vi "Analyse.vi"(8 "error in (no error)":errorcluster, 10 "ImageData":T1, 11 "FluorescenceAnalyser in":refnum<class "FluorescenceAnalyser.lvclass">) -> (0 "error out":errorcluster, 3 "FluorescenceAnalyser out":refnum<class "FluorescenceAnalyser.lvclass">)   [LabVIEW 2009, in "Tools.lvlib" / "Imaging.lvlib" / "FluorescenceAnalyser.lvclass"]
uses:
  FluorescenceAnalyser.lvclass
  ImageAnalyser.lvclass
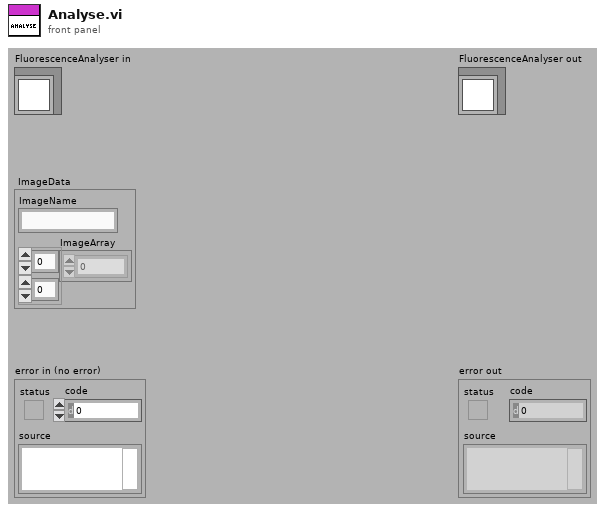
[diagram p1: front panel]
types:
  T1 = cluster{"ImageName":string, "ImageArray":sgl[][]}
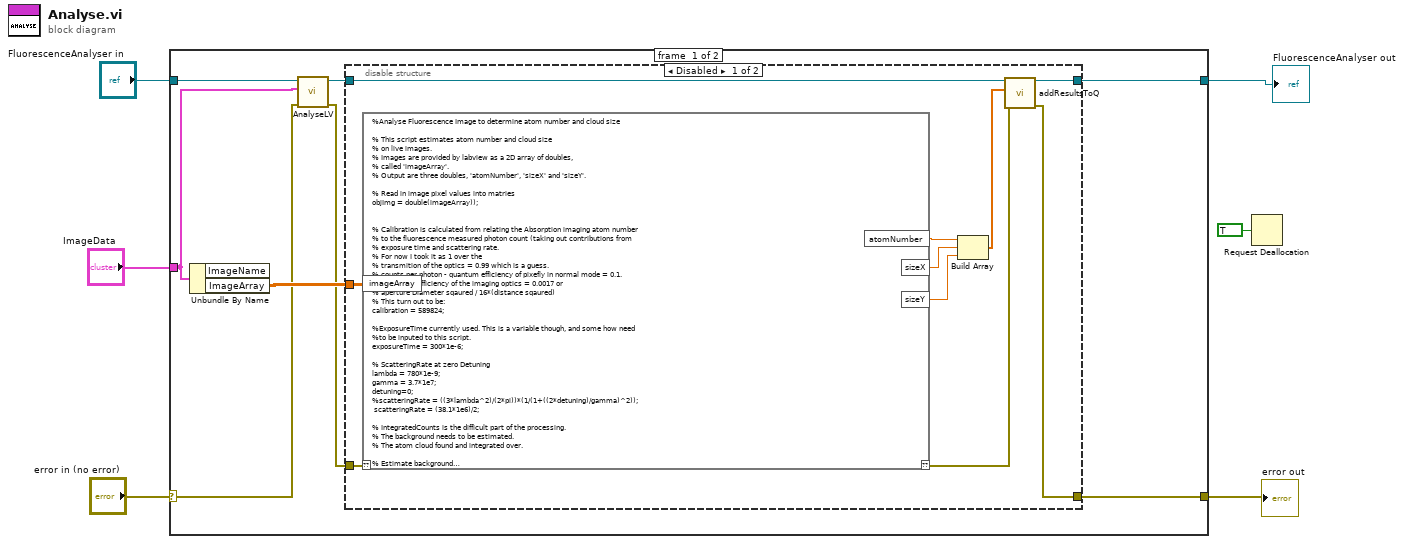
[diagram p0: block diagram]
diagram:
  n1 = case shown="No Error" "error in (no error)" {
    selector: "error in (no error)" -> [w8 w27]
    tunnel: "FluorescenceAnalyser in" -> [w11 w28]
    tunnel: "ImageData" -> [w10 _]
    tunnel: [w12 w27] -> w3
    tunnel: [w13 w28] -> w2
    frame #0 {
      n2 = Unbundle By Name(w10) -> ("ImageArray"=w14:sgl[][])  [unwired: 1 out]
      n3 = call "AnalyseLV.vi"("error in (no error)"=w8, "ImageData"=w10, "FluorescenceAnalyser in"=w11) -> ("error out"=w7:errorcluster, "FluorescenceAnalyser out"=w9:refnum<class "FluorescenceAnalyser.lvclass">)  [unwired: 7 in]
      n4 = disable-structure shown="Disabled" {
        disable-tunnel: w14 -> [w24 _]
        disable-tunnel: [w20 w26] -> w13
        disable-tunnel: [w19 w25] -> w12
        disable-tunnel: w7 -> [w17 w25]
        disable-tunnel: w9 -> [w16 w26]
        frame #0 {
          n5 = script code="%Analyse Fluorescence Image to determine atom number and cloud size\n\n% This script estimates atom number and cloud size\n% on live images. \n% Images are provided by labview as a 2D array of doubles,\n% called 'imageArray'.\n% Output are three doubles, 'atomNumber', 'sizeX' and 'sizeY'.\n\n% Read in image pixel values into matries\nobjImg = double(imageArray));\n\n\n% Calibration is calculated from relating the Absorption imaging atom number\n% to the fluorescence measured photon count (taking out contributions from\n% exposure time and scattering rate.\n% For now I took it as 1 over the \n% transmition of the optics = 0.99 which is a guess.\n% counts per photon - quantum efficiency of pixefly in normal mode = 0.1.\n% Collection efficiency of the imaging optics = 0.0017 or \n% aperture Diameter sqaured / 16*(distance sqaured)\n% This turn out to be:\ncalibration = 589824;\n\n%ExposureTime currently used. This is a variable though, and some how need\n%to be inputed to this script.\nexposureTime = 300*1e-6;\n\n% ScatteringRate at zero Detuning\nlambda = 780*1e-9;\ngamma = 3.7*1e7;\ndetuning=0;\n%scatteringRate = ((3*lambda^2)/(2*pi))*(1/(1+((2*detuning)/gamma)^2));\n scatteringRate = (38.1*1e6)/2;\n\n% IntegratedCounts is the difficult part of the processing.\n% The background needs to be estimated.\n% The atom cloud found and integrated over.\n\n% Estimate background \nbg = mean(mean(objImg(10,:)));\n\nimage = objImg-bg;\n\nintegratedCounts = sum(sum(image));\n%absimagecount=integratedCounts*scatteringRate/(6.45e-6)^2;\n%Calculate Atom number\natomNumber = ( calibration/(exposureTime*scatteringRate) )*integratedCounts;\n\n%subplot(3,2,1), imagesc(image(200:800,400:1000)), \n%subplot(3,2,2), plot(image(:,691));\n%subplot(3,2,3), plot(image(507,:));\n%axes('position',[0,0,1,1],'visible','off');\n%text(.5,.25,['Atom Number = ',num2str(atomNumber/10^9),' x 10^9']);\n\n\n% gaussian distribution in x direction\nxdata1=sum(image,1);\n\nX1=1:length(xdata1);\nY1=xdata1(X1);\n\n[maxValue1,maxIndex1] = max(xdata1);\ninitialCoeff1 = [0,max(xdata1)-min(xdata1),maxIndex1,60];\n\noptions = optimset('Largescale','off');\n    \nx1=lsqnonlin(@fit_simp,initialCoeff1,[],[],options,X1,Y1);\n\nY1_new = x1(1) + x1(2)*exp(-0.5*((X1-x1(3))/x1(4)).^2);\n\n% gaussian distribution in y direction\nxdata2=sum(image,2);\nxdata2=xdata2';\n\nX2=1:length(xdata2);\nY2=xdata2(X2);\n\n[maxValue2,maxIndex2] = max(xdata2);\ninitialCoeff2 = [0,max(xdata2)-min(xdata2),maxIndex2,60];\n\noptions = optimset('Largescale','off');\n    \nx2=lsqnonlin(@fit_simp,initialCoeff2,[],[],options,X2,Y2);\n\nY2_new = x2(1) + x2(2)*exp(-0.5*((X2-x2(3))/x2(4)).^2);\n\n%plot fits\n%figure, plot(X2,Y2,'+r',X2,Y2_new,'b');\n%figure, plot(X1,Y1,'+r',X1,Y1_new,'b');\n\n\n% Find cloud size in mm\npixelSize = 6.45*1e-6;\nsizeX = x1(4)*(2*sqrt(log(2)))*pixelSize*1000;\nsizeY = x2(4)*(2*sqrt(log(2)))*pixelSize*1000;"("??"=w17, "imageArray"=w24) -> ("??"=w18:errorcluster, "atomNumber"=w23:dbl, "sizeX"=w22:dbl, "sizeY"=w21:dbl)
          n6 = Build Array(w23, w22, w21) -> (w15:dbl[])
          n7 = call "addResultsToQ.vi"("error in (no error)"=w18, "Results"=w15, "ImageAnalyser in"=w16) -> ("error out"=w19:errorcluster, "ImageAnalyser out"=w20:refnum<class "FluorescenceAnalyser.lvclass">)  [unwired: 7 in]
        }
        frame #1 {
        }
      }
    }
    frame #1 {
    }
  }
  "error out" <- w3
  "FluorescenceAnalyser out" <- w2
  n8 = Request Deallocation(TRUE ("flag")) -> ()
